vi "DM Pixel Scan Counter.vi"(0 "Initial Mirror Modes":T1, 2 "Action":T2, 7 "Pixel Scan Parameters In":T3={"Scan Start Pixel"=1, "Scan End Pixel"=1, "Pixel Start Value (-1 to 1)"=-0.5, "Pixel End Value (-1 to 1)"=0.5, "Number of Steps"=0.1}, 11 "Initial Pixel Values (-1 to 1)":dbl[](array[numeric])) -> (4 "Scan Done":bool, 6 "DM Pixel":i32, 10 "Normalized DM Pixel Value":dbl, 13 "Initial Mirror Modes OUT":T1, 15 "Initial Pixel Values OUT":dbl[](array[numeric]))   [LabVIEW 2016]
uses:
  Controls/Pixel Scan Parameters.ctl
  Controls/Standard_Counter_Action.ctl
  Controls/MirrorModes.ctl
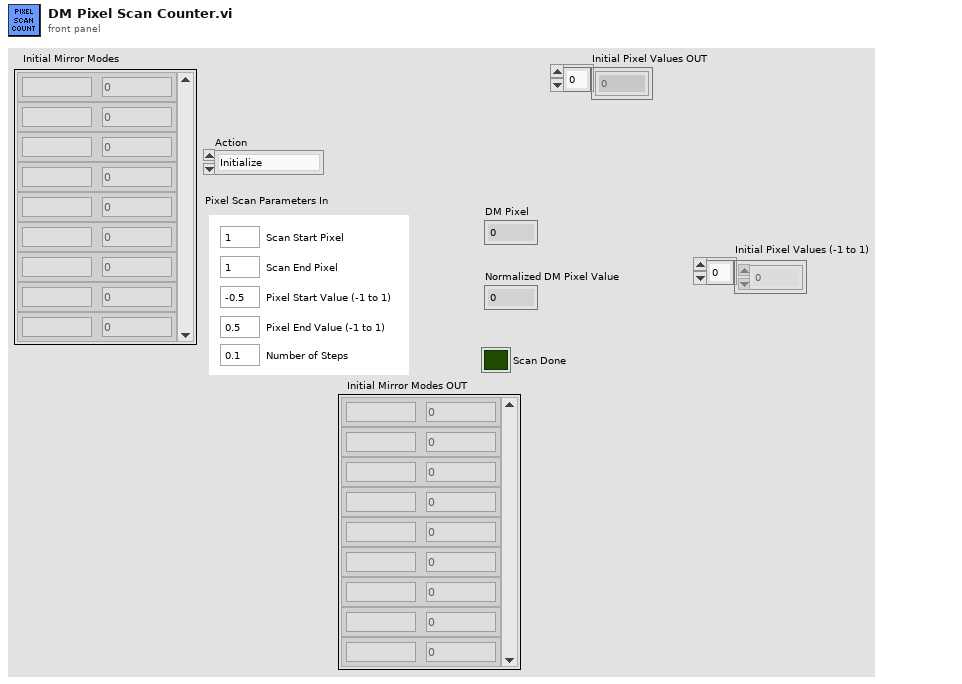
[diagram p1: front panel]
types:
  T1 = typedef "MirrorModes.ctl" = cluster{"Mode":string, "Amplitude":dbl}[]
  T2 = typedef "Standard_Counter_Action.ctl" = enum16{"Initialize", "Update Count", "Get Count"}
  T3 = typedef "Pixel Scan Parameters.ctl" = cluster{"Scan Start Pixel":i32, "Scan End Pixel":i32, "Pixel Start Value (-1 to 1)":dbl, "Pixel End Value (-1 to 1)":dbl, "Number of Steps":dbl}
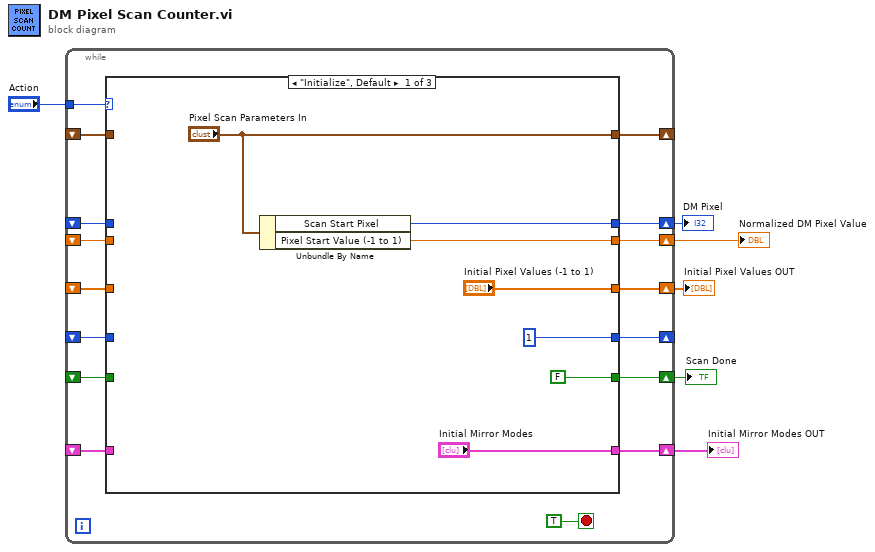
[diagram p0: block diagram]
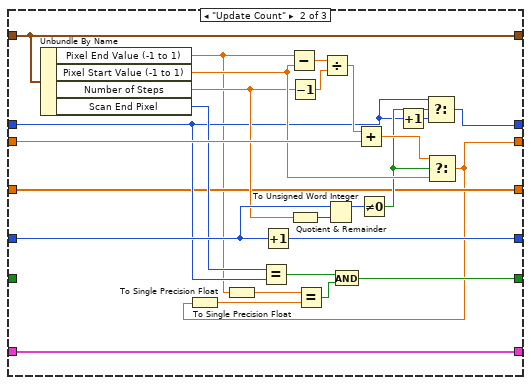
[diagram p2: hidden frame]
diagram:
  n1 = while {
    tunnel: "Action" -> [w21]
    shift-right: [w20] -> _
    shift-left: _ -> [w15]
    shift-right: [w19] -> w3
    shift-left: _ -> [w17]
    shift-right: [w18] -> w2
    shift-left: _ -> [w16]
    shift-right: [w14] -> _
    shift-left: _ -> [w13]
    shift-right: [w12] -> w5
    shift-left: _ -> [w11]
    shift-right: [w10] -> w4
    shift-left: _ -> [w9]
    shift-right: [w8] -> w1
    shift-left: _ -> [w7]
    stop <- TRUE stop-if-true
    n2 = case shown="\"Initialize\", Default" w21 {
      tunnel: ["Pixel Scan Parameters In" w54 w60] -> w20
      tunnel: [w28 w41 w62] -> w19
      tunnel: [w27 w31 w61] -> w18
      tunnel: w17 -> [_ w36 w62]
      tunnel: w16 -> [_ w52 w61]
      tunnel: w15 -> [_ w54 w60]
      tunnel: [u16 1 w49 w59] -> w14
      tunnel: w13 -> [_ w51 w59]
      tunnel: [FALSE w37 w58] -> w12
      tunnel: w11 -> [_ _ w58]
      tunnel: ["Initial Pixel Values (-1 to 1)" w35 w57] -> w10
      tunnel: w9 -> [_ w35 w57]
      tunnel: ["Initial Mirror Modes" w30 w56] -> w8
      tunnel: w7 -> [_ w30 w56]
      frame "Initialize", Default {
        n3 = Unbundle By Name("Pixel Scan Parameters In") -> ("Scan Start Pixel"=w28:i32, "Pixel Start Value (-1 to 1)"=w27:dbl)
      }
      frame "Update Count" {
        n4 = Unbundle By Name(w54) -> ("Pixel End Value (-1 to 1)"=w34:dbl, "Pixel Start Value (-1 to 1)"=w47:dbl, "Number of Steps"=w45:dbl, "Scan End Pixel"=w40:i32)
        n5 = To Single Precision Float(number=w34) -> (single precision float=w33:sgl)
        n6 = Equal?(x=w40, y=w36) -> (x = y?=w39:bool)
        n7 = Increment(x=w51) -> (x+1=w49:u16)
        n8 = Subtract(x=w34, y=w47) -> (x-y=w55:dbl)
        n9 = Decrement(x=w45) -> (x-1=w44:dbl)
        n10 = To Unsigned Word Integer(number=w45) -> (unsigned 16bit integer=w50:u16)
        n11 = Divide(x=w55, y=w44) -> (x/y=w53:dbl)
        n12 = Quotient & Remainder(x=w51, y=w50) -> (x-y*floor(x/y)=w48:u16)  [unwired: 1 out]
        n13 = Add(x=w53, y=w52) -> (x+y=w46:dbl)
        n14 = Not Equal To 0?(x=w48) -> (x != 0?=w43:bool)
        n15 = Increment(x=w36) -> (x+1=w42:i32)
        n16 = Select(t=w36, s=w43, f=w42) -> (s? t:f=w41:i32)
        n17 = Select(t=w46, s=w43, f=w47) -> (s? t:f=w31:dbl)
        n18 = To Single Precision Float(number=w31) -> (single precision float=w32:sgl)
        n19 = Equal?(x=w33, y=w32) -> (x = y?=w38:bool)
        n20 = And(x=w39, y=w38) -> (x .and. y?=w37:bool)
      }
      frame "Get Count" {
      }
    }
  }
  "DM Pixel" <- w3
  "Normalized DM Pixel Value" <- w2
  "Scan Done" <- w5
  "Initial Pixel Values OUT" <- w4
  "Initial Mirror Modes OUT" <- w1
